vi "TypeOfHexaboardVi.vi"(11 "Type of Hexaboard":T1) -> ()   [LabVIEW 2021]
uses:
  TypeOfHexaboard.ctl
  Routine.lvclass
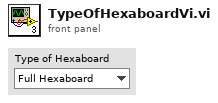
[diagram p1: front panel]
types:
  T1 = typedef "Routine.lvclass/TypeOfHexaboard.ctl" = enum16{"Full Hexaboard", "Right Partial"}
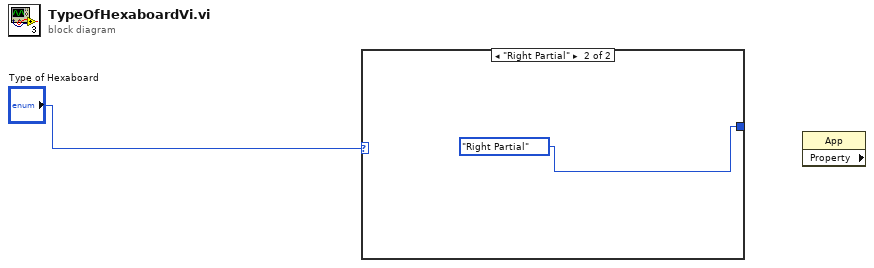
[diagram p0: block diagram]
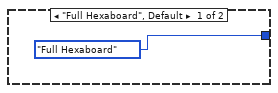
[diagram p2: hidden frame]
diagram:
  n1 = case shown="\"Right Partial\"" "Type of Hexaboard" {
    tunnel: [TypeOfHexaboard."Full Hexaboard" ("Type of Hexaboard") TypeOfHexaboard."Right Partial" ("Type of Hexaboard")] -> _
    frame "Full Hexaboard", Default {
    }
    frame "Right Partial" {
    }
  }
  n2 = property class="App" props=[]() -> ()  [unwired: 2 in, 3 out]
